vi "Calculate X Y Waveform Voltage Out Whole Image.vi"(7 "Raster Scan Direction":T1, 8 "Y Flyback":dbl[][](graph), 9 "Y Waveform":dbl[](graph), 10 "X Flyback":dbl[][](graph), 11 "X Waveform":dbl[](graph)) -> (1 "Y Waveform Out":dbl[](graph), 2 "DO":i16[](graph), 3 "X Waveform Out":dbl[](graph), 4 "Digital Line Acq":bool[](array[boolean]), 5 "XY Waveform Out":dbl[][](graph))   [LabVIEW 2018]
uses:
  Controls/Scan Direction.ctl
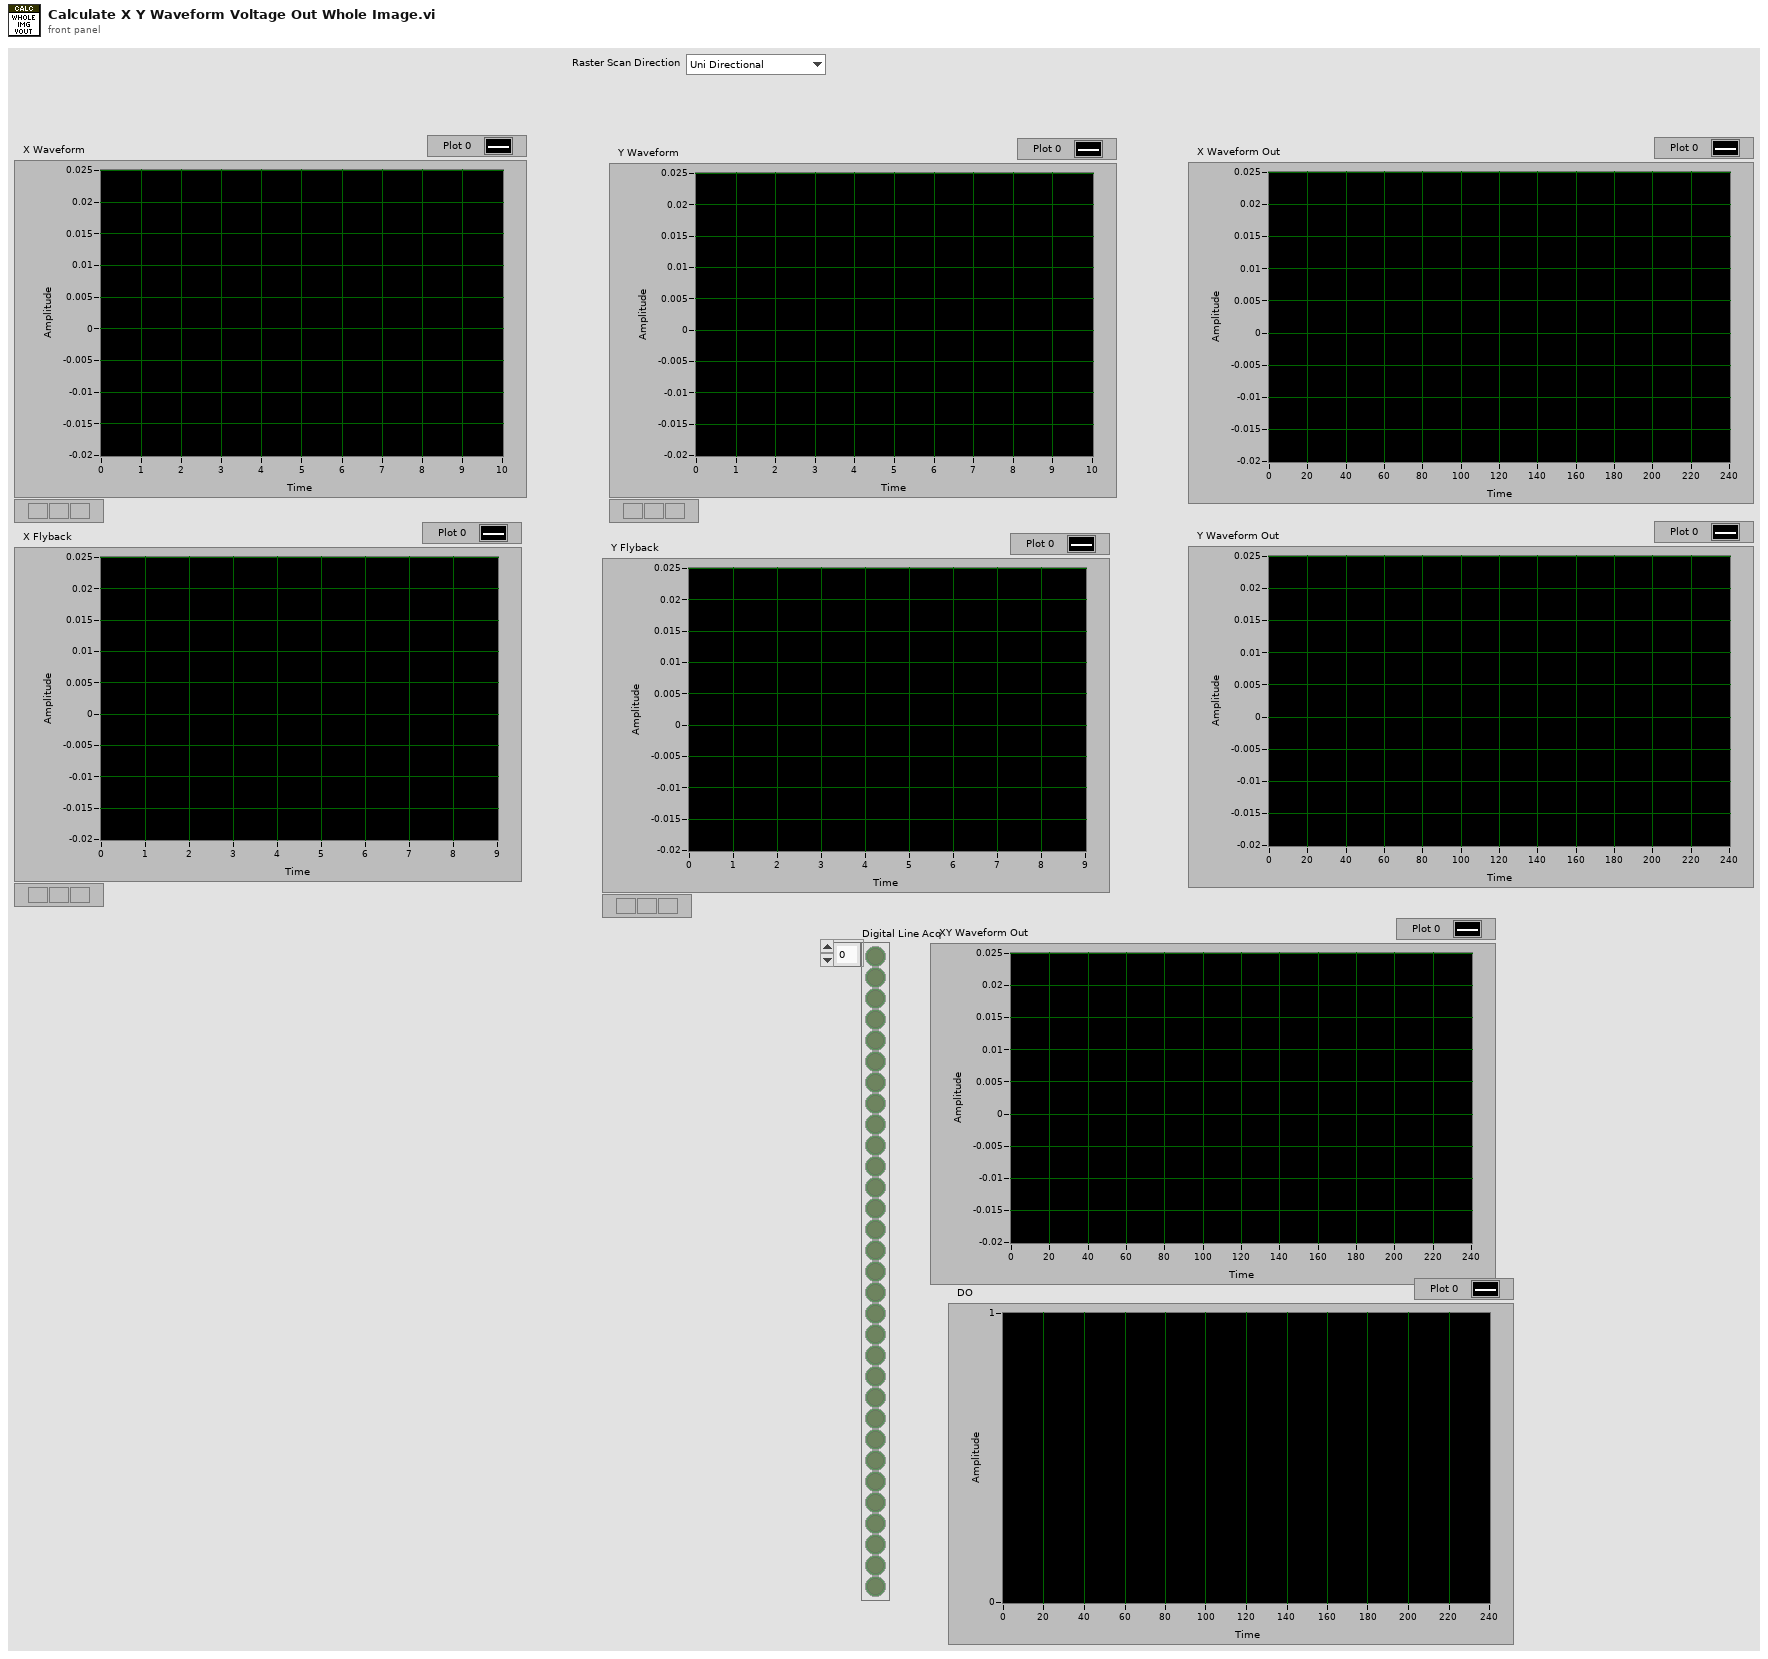
[diagram p1: front panel]
types:
  T1 = typedef "Scan Direction.ctl" = enum16{"Uni Directional", "Bi Directional", "None"}
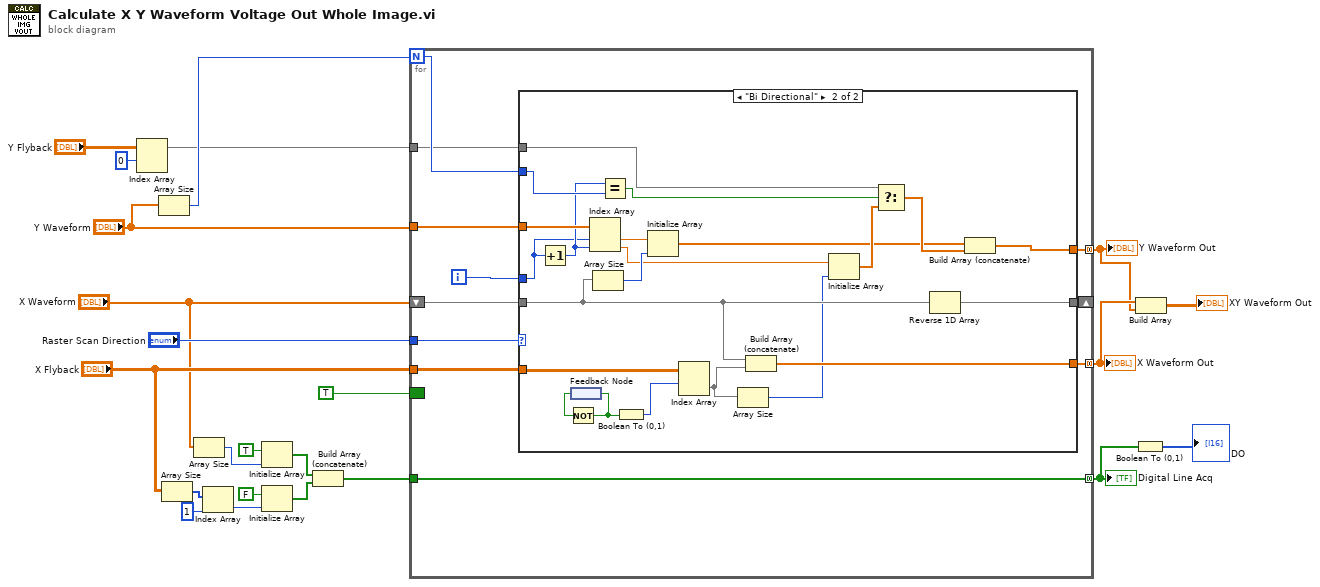
[diagram p0: block diagram]
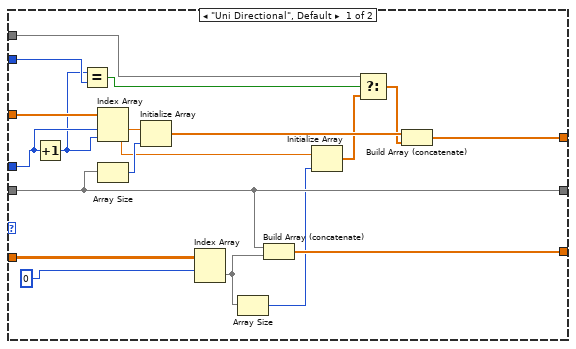
[diagram p2: hidden frame]
diagram:
  n1 = Index Array(array="Y Flyback", index (row)=0) -> (element=w19:dbl[])  [unwired: 1 in]
  n2 = Array Size(array="Y Waveform") -> (size(s)=w21:i32)
  n3 = Array Size(array="X Flyback") -> (size(s)=w12:i32[])
  n4 = Array Size(array="X Waveform") -> (size(s)=w7:i32)
  n5 = Index Array(array=w12, index=1) -> (element=w11:i32)
  n6 = Initialize Array(TRUE, w7) -> (w6:bool[])
  n7 = Initialize Array(FALSE, w11) -> (w5:bool[])
  n8 = Build Array (concatenate)(w6, w5) -> (w4:bool[])
  n9 = for {
    N: w21 -> [w26]
    shift-right: [w34] -> _
    shift-left: "X Waveform" -> [w33]
    tunnel: "Raster Scan Direction" -> [w32]
    tunnel: "Y Waveform" -> [w28]
    tunnel: "X Flyback" -> [w31]
    tunnel: [w29] -> w17 mode=concatenating
    tunnel: [w27] -> w16 mode=concatenating
    tunnel: w19 -> [w25]
    border: TRUE -> [_]
    tunnel: w4 -> [w24]
    tunnel: [w24] -> w1 mode=concatenating
    i -> [w30]
    n10 = case shown="\"Bi Directional\"" w32 {
      tunnel: [w47 w75] -> w34
      tunnel: w33 -> [w47 w65]
      tunnel: w31 -> [w53 w74]
      tunnel: w30 -> [w41 w67]
      tunnel: [w51 w73] -> w29
      tunnel: w28 -> [w50 w69]
      tunnel: [w42 w58] -> w27
      tunnel: w26 -> [w40 w70]
      tunnel: w25 -> [w36 w71]
      frame "Uni Directional", Default {
        n11 = Increment(x=w41) -> (x+1=w35:i32)
        n12 = Equal?(x=w35, y=w40) -> (x = y?=w39:bool)
        n13 = Index Array(array=w50, index #1=w41, index #2=w35) -> (element #1=w49:dbl, element #2=w46:dbl)
        n14 = Array Size(array=w47) -> (size(s)=w48:i32)
        n15 = Initialize Array(w49, w48) -> (w43:dbl[])
        n16 = Index Array(array=w53, index (row)=0 ("disabled index (col)")) -> (element=w45:dbl[])  [unwired: 1 in]
        n17 = Array Size(array=w45) -> (size(s)=w44:i32)
        n18 = Build Array (concatenate)(w47, w45) -> (w51:dbl[])
        n19 = Initialize Array(w46, w44) -> (w37:dbl[])
        n20 = Select(t=w36, s=w39, f=w37) -> (s? t:f=w38:dbl[])
        n21 = Build Array (concatenate)(w43, w38) -> (w42:dbl[])
      }
      frame "Bi Directional" {
        n22 = Increment(x=w67) -> (x+1=w68:i32)
        n23 = feedback #1() -> (w56:bool)
        n24 = Not(x=w56) -> (.not. x?=w55:bool)
        n25 = feedback-in #1(w55) -> ()
        n26 = Index Array(array=w69, index #1=w67, index #2=w68) -> (element #1=w66:dbl, element #2=w63:dbl)
        n27 = Array Size(array=w65) -> (size(s)=w64:i32)
        n28 = Equal?(x=w68, y=w70) -> (x = y?=w72:bool)
        n29 = Boolean To (0,1)(Boolean=w55) -> (0, 1=w54:i16)
        n30 = Initialize Array(w66, w64) -> (w57:dbl[])
        n31 = Index Array(array=w74, index (row)=w54) -> (element=w61:dbl[])  [unwired: 1 in]
        n32 = Array Size(array=w61) -> (size(s)=w60:i32)
        n33 = Build Array (concatenate)(w65, w61) -> (w73:dbl[])
        n34 = Initialize Array(w63, w60) -> (w62:dbl[])
        n35 = Select(t=w71, s=w72, f=w62) -> (s? t:f=w59:dbl[])
        n36 = Reverse 1D Array(array=w65) -> (reversed array=w75:dbl[])
        n37 = Build Array (concatenate)(w57, w59) -> (w58:dbl[])
      }
    }
  }
  "X Waveform Out" <- w17
  "Y Waveform Out" <- w16
  "Digital Line Acq" <- w1
  n38 = Boolean To (0,1)(Boolean=w1) -> (0, 1=→"DO":i16[])
  n39 = Build Array(w17, w16) -> (→"XY Waveform Out":dbl[][])
